vi "Lectura de datos.vi"() -> ()   [LabVIEW 2020]
panel:
  in  "stop":bool
  out "Grafico señal":dynamicdata(graph)
  out "Lim":dbl
  out "Alarma":bool
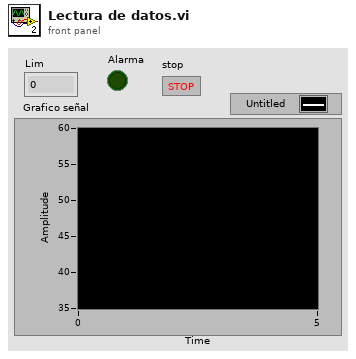
[diagram p1: front panel]
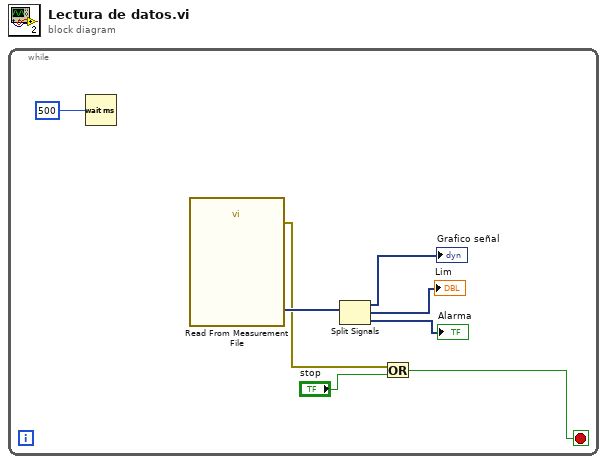
[diagram p0: block diagram]
diagram:
  n1 = while {
    stop <- w4 stop-if-true
    n2 = Wait (ms)(milliseconds to wait=u32 500 ("millisecond timer value")) -> ()  [unwired: 1 out]
    n3 = call "Read From Measurement File"() -> ("error out"=w6:errorcluster, "Signals"=w7:dynamicdata)  [unwired: 6 in, 4 out]
    n4 = Split Signals(w7) -> (→"Grafico señal":dynamicdata, →"Lim":dynamicdata, →"Alarma":dynamicdata)  [unwired: 3 in]
    n5 = Or(x=w6, y="stop") -> (x .or. y?=w4:bool)
  }
